vi "Main UI.vi"(8 "error in (no error)":errorcluster, 11 "SB App in":refnum<class "SB App.lvclass">) -> (0 "error out":errorcluster, 3 "SB App out":refnum<class "SB App.lvclass">)   [LabVIEW 2020, in "SB App.lvlib" / "SB App.lvclass"]
uses:
  SB App.lvclass
  Display Mode.ctl
  SB App.lvclass/SB App.ctl
  Incoming Events.ctl
  Board Size Update.ctl
  Game Start Data.ctl
  SquareBattle/Team Start Info.ctl
  SquareBattle/Team/Team.lvclass
  SquareBattle/Position.ctl
  Start Position Data.ctl
  SquareBattle/Team ID.ctl
  SB App.lvlib
  SquareBattle/SquareBattle.lvlib
  SquareBattle/Game/Game.lvclass
  Game Config Panel/Game Config Panel.lvclass
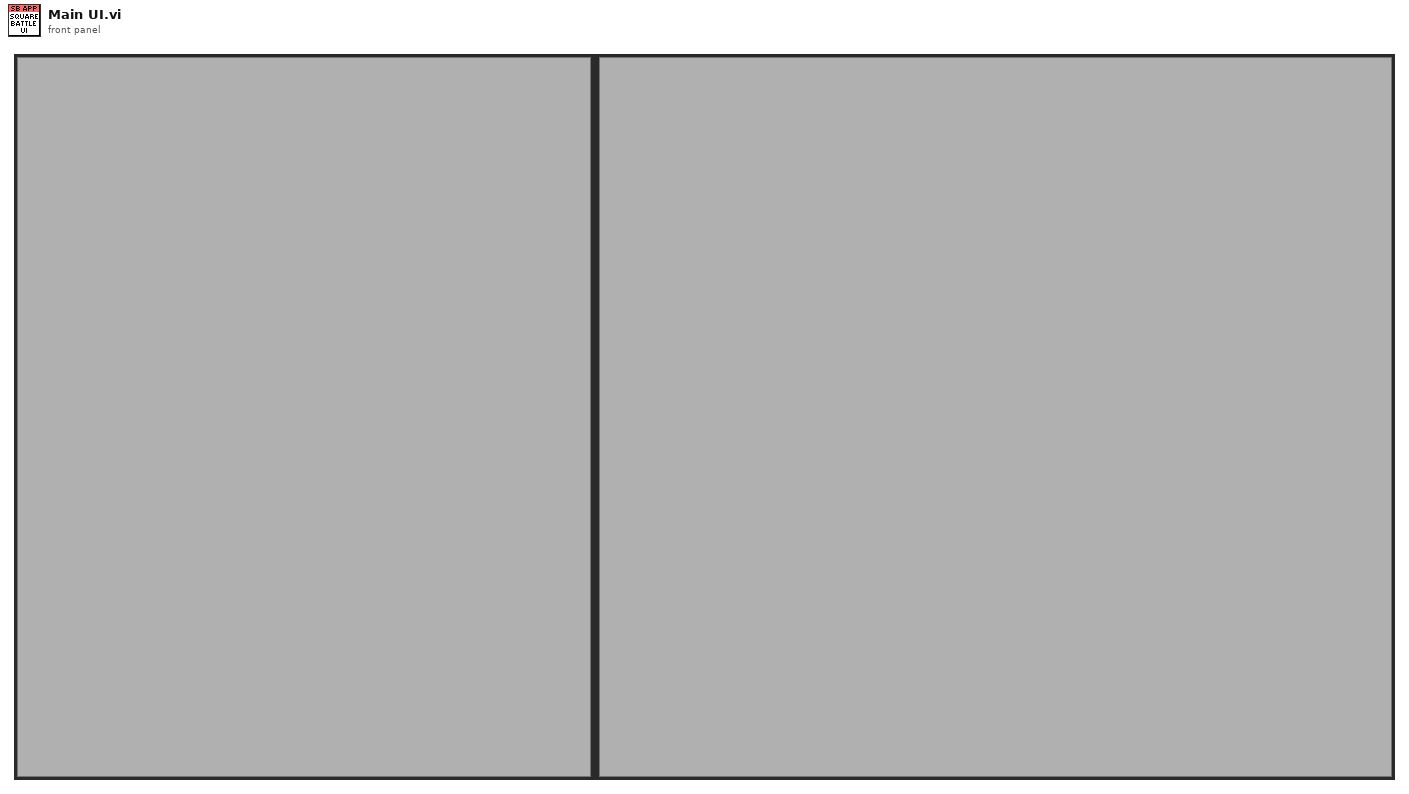
[diagram p1: front panel]
types:
  T1 = enum32{"Invalid", "Standard", "Closed", "Hidden", "Minimized", "Maximized"}
  T2 = typedef "SB App.lvlib/Display Mode.ctl" = enum16{"Config", "Team", "Squares", "Done"}
  T3 = typedef "SB App.lvlib/SB App.lvclass/Incoming Events.ctl" = cluster{"Board Size Update":refnum<user-event>, "Game Start":refnum<user-event>, "Add Team":refnum<user-event>, "Remove Team":refnum<user-event>, "Start Position":refnum<user-event>}
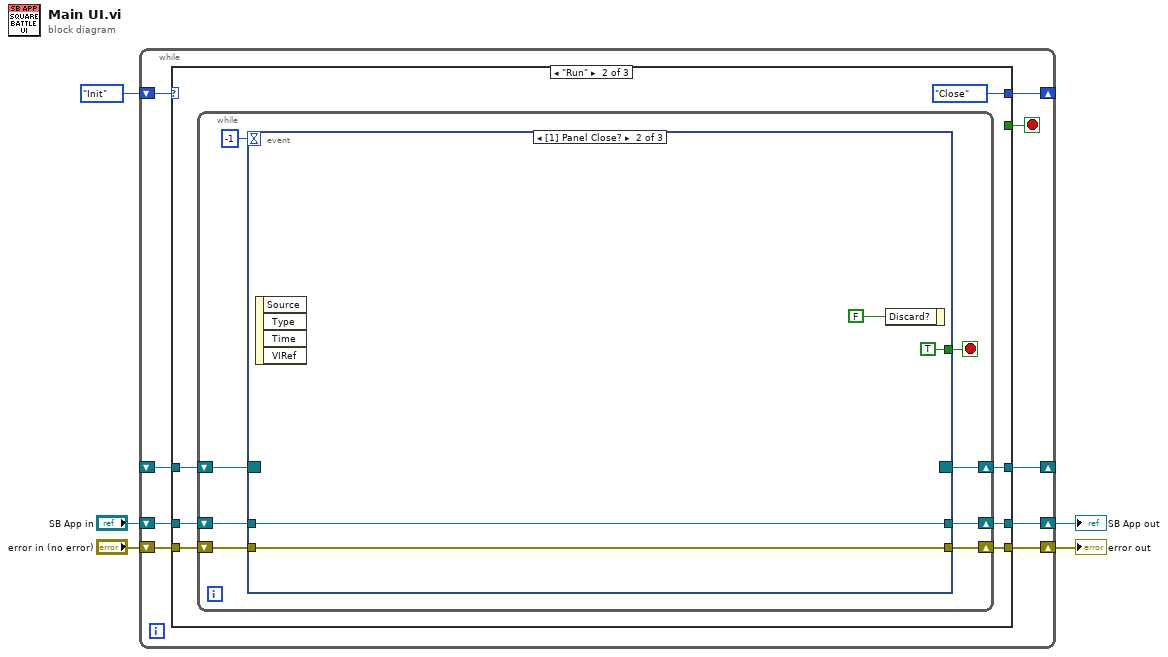
[diagram p0: block diagram]
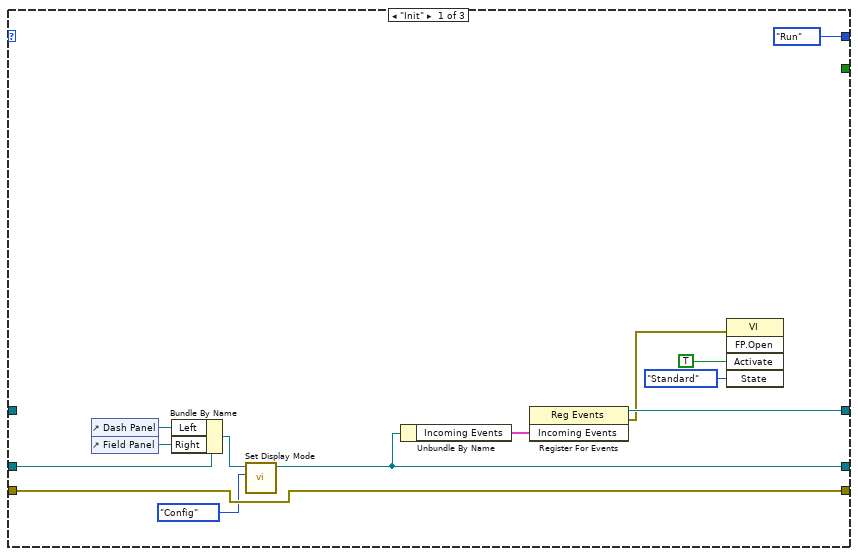
[diagram p2: hidden frame]
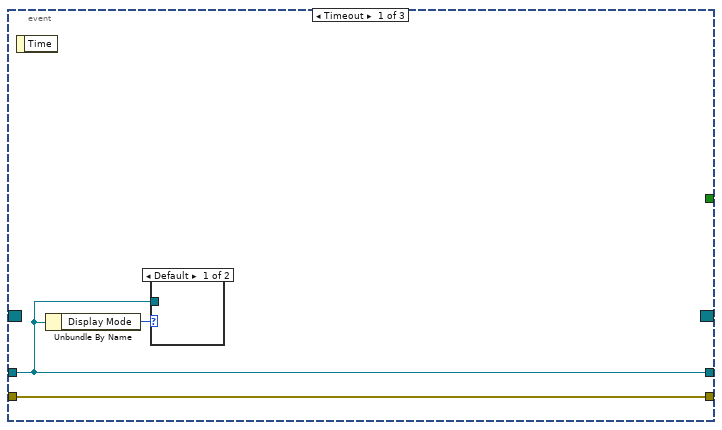
[diagram p3: hidden frame]
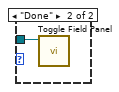
[diagram p4: hidden frame]
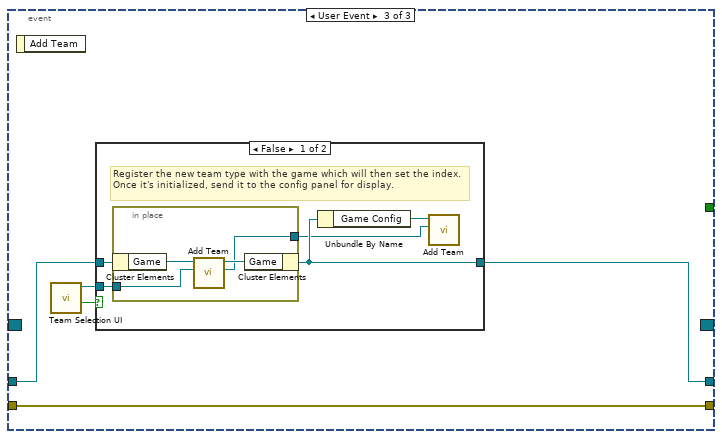
[diagram p5: hidden frame]
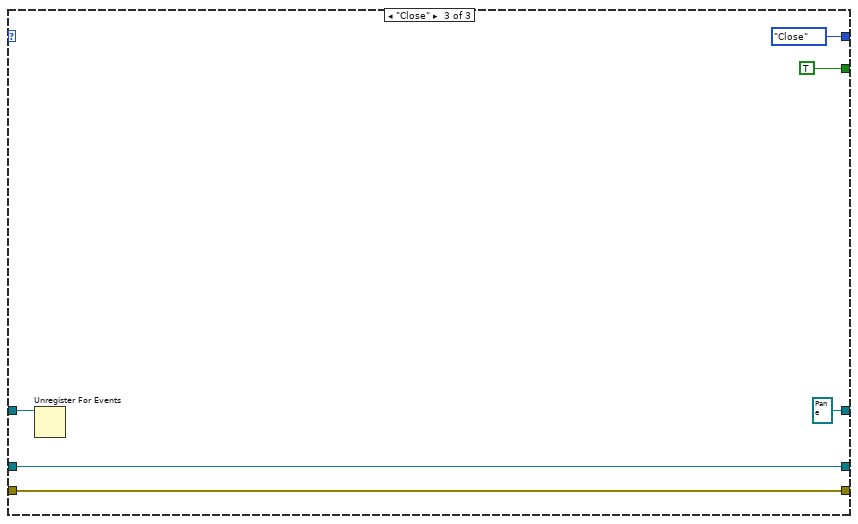
[diagram p7: hidden frame]
diagram:
  n1 = while {
    shift-right: [w13] -> _
    shift-left: enum16{"Init", "Run", "Close"}."Init" ("Basic UI State") -> [w14]
    shift-right: [w8] -> w2
    shift-left: "SB App in" -> [w12]
    shift-right: [w9] -> w1
    shift-left: "error in (no error)" -> [w11]
    shift-right: [w7] -> _
    shift-left: _ -> [w6]
    stop <- w10 stop-if-true
    n2 = case shown="\"Run\"" w14 {
      tunnel: [enum16{"Init", "Run", "Close"}."Run" ("Basic UI State") enum16{"Init", "Run", "Close"}."Close" ("Basic UI State") enum16{"Init", "Run", "Close"}."Close" ("Basic UI State")] -> w13
      tunnel: w12 -> [w26 w33 w69]
      tunnel: w11 -> [w20 w32 w68]
      tunnel: [_ _ TRUE] -> w10
      tunnel: [w20 w30 w68] -> w9
      tunnel: [w18 w31 w69] -> w8
      tunnel: [w22 w28 refnum<event-registration> refnum ("Event Registration Refnum")] -> w7
      tunnel: w6 -> [_ w29 w67]
      frame "Init" {
        n3 = control-ref of="Dash Panel"() -> (w25:refnum<vi>)
        n4 = control-ref of="Field Panel"() -> (w24:refnum<vi>)
        n5 = Bundle By Name(cluster=w26, "Left"=w25, "Right"=w24) -> (w19:refnum<class "SB App.lvclass">)
        n6 = call "Set Display Mode.vi"("Display Mode"=Display_Mode."Config", "SB App in"=w19) -> ("SB App out"=w18:refnum<class "SB App.lvclass">)  [unwired: 9 in]
        n7 = Unbundle By Name(w18) -> ("Incoming Events"=w23:T3)
        n8 = register-events(w23) -> (reference out=w22:refnum<event-registration>, error out=w21:errorcluster)  [unwired: 2 in]
        n9 = invoke class="VI" method="FP.Open"(error in=w21, "Activate"=TRUE ("Activate?"), "State"=T1."Standard") -> ()  [unwired: 2 in, 5 out]
      }
      frame "Run" {
        n10 = while {
          shift-right: [w39] -> w31
          shift-left: w33 -> [w42]
          shift-right: [w38] -> w30
          shift-left: w32 -> [w41]
          shift-right: [w35] -> w28
          shift-left: w29 -> [w36]
          stop <- w40 stop-if-true
          n11 = event shown="[1] Panel Close?" {
            selector: w36 -> [_ _ _]
            dyn-events: [_ _ _] -> w35
            timeout: -1 -> [_ _ _]
            tunnel: w42 -> [w43 w50 w54]
            tunnel: w41 -> [w45 w49 w55]
            tunnel: [_ TRUE ("Discard?") _] -> w40
            tunnel: [w43 w50 w51] -> w39
            tunnel: [w45 w49 w55] -> w38
            event Timeout {
              n12 = event-data() -> ()  [unwired: 1 in, 1 out]
              n13 = Unbundle By Name(w43) -> ("Display Mode"=w44:T2)
              n14 = case shown="Default" w44 {
                tunnel: w43 -> [_ w46]
                frame Default {
                }
                frame "Done" {
                  n15 = call "Toggle Field Panel.vi"("SB App in"=w46) -> ()  [unwired: 9 in, 2 out]
                }
              }
            }
            event Panel Close? {
              n16 = event-data() -> ()  [unwired: 1 in, 4 out]
              n17 = event-data("Discard?"=FALSE) -> ()  [unwired: 1 in, 1 out]
            }
            event User Event {
              n18 = event-data() -> ()  [unwired: 1 in, 1 out]
              n19 = call "Team Selection UI.vi"() -> ("Cancelled"=w52:bool, "Team"=w53:refnum<class "Team.lvclass">)  [unwired: 10 in]
              n20 = case shown="False" w52 {
                tunnel: w54 -> [w60 w65]
                tunnel: w53 -> [w59 _]
                tunnel: [w58 w65] -> w51
                frame False {
                  # "Register the new team type with the game which will then set the index. Once it's initialized, send it to the config panel for display."
                  n21 = in-place {
                    in-place-border: w59 -> [w63]
                    in-place-border: [w61] -> w56
                    n22 = in-place-cluster #1(w60) -> ("Game"=w64:refnum<class "Game.lvclass">)
                    n23 = call "Add Team.vi"("Team Type"=w63, "Game in"=w64) -> ("Team"=w61:refnum<class "Team.lvclass">, "Game out"=w62:refnum<class "Game.lvclass">)  [unwired: 7 in, 1 out]
                    n24 = in-place-cluster #1("Game"=w62) -> (w58:refnum<class "SB App.lvclass">)
                  }
                  n25 = Unbundle By Name(w58) -> ("Game Config"=w57:refnum<class "Game Config Panel.lvclass">)
                  n26 = call "Add Team.vi"("Team"=w56, "Game Config Panel in"=w57) -> ()  [unwired: 8 in, 2 out]
                }
                frame True {
                  # "User cancelled selection, don't need to do anything."
                }
              }
            }
          }
        }
      }
      frame "Close" {
        n27 = Unregister For Events(event registration refnum=w67) -> ()  [unwired: 1 in, 1 out]
      }
    }
  }
  "error out" <- w1
  "SB App out" <- w2
